vi "FTW-CodeGen-FindGObjectTaggedForScripting.vi"(0 "GObject to Traverse":refnum<vi>, 5 "Class Name":string="GObject", 7 "Label to uniquely identify node":string="#FTW-CodeGen", 11 "error in":errorcluster) -> (6 "GObject":refnum<vi>, 15 "error out":errorcluster)   [LabVIEW 2013, in "Featherweight.lvlib" / "FTW-CodeGen.lvlib"]
uses:
  FTW-CodeGen.lvlib
  Featherweight.lvlib
panel:
  # "Inputs"
  # "Outputs"
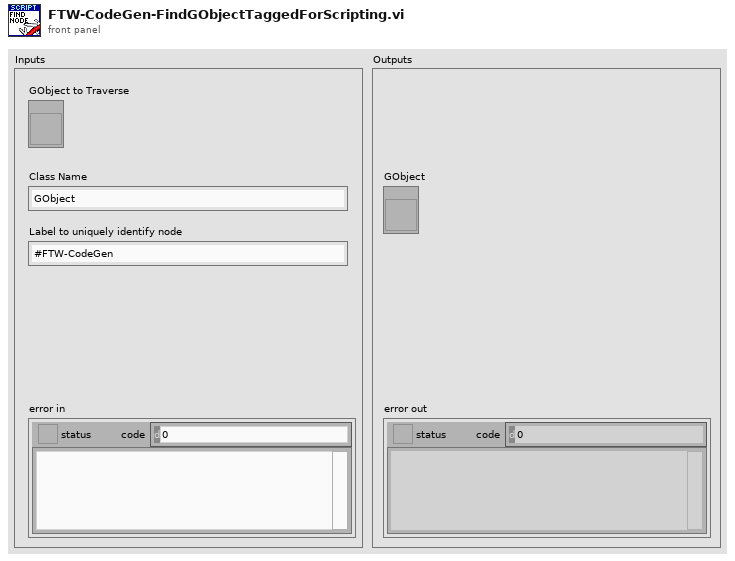
[diagram p1: front panel]
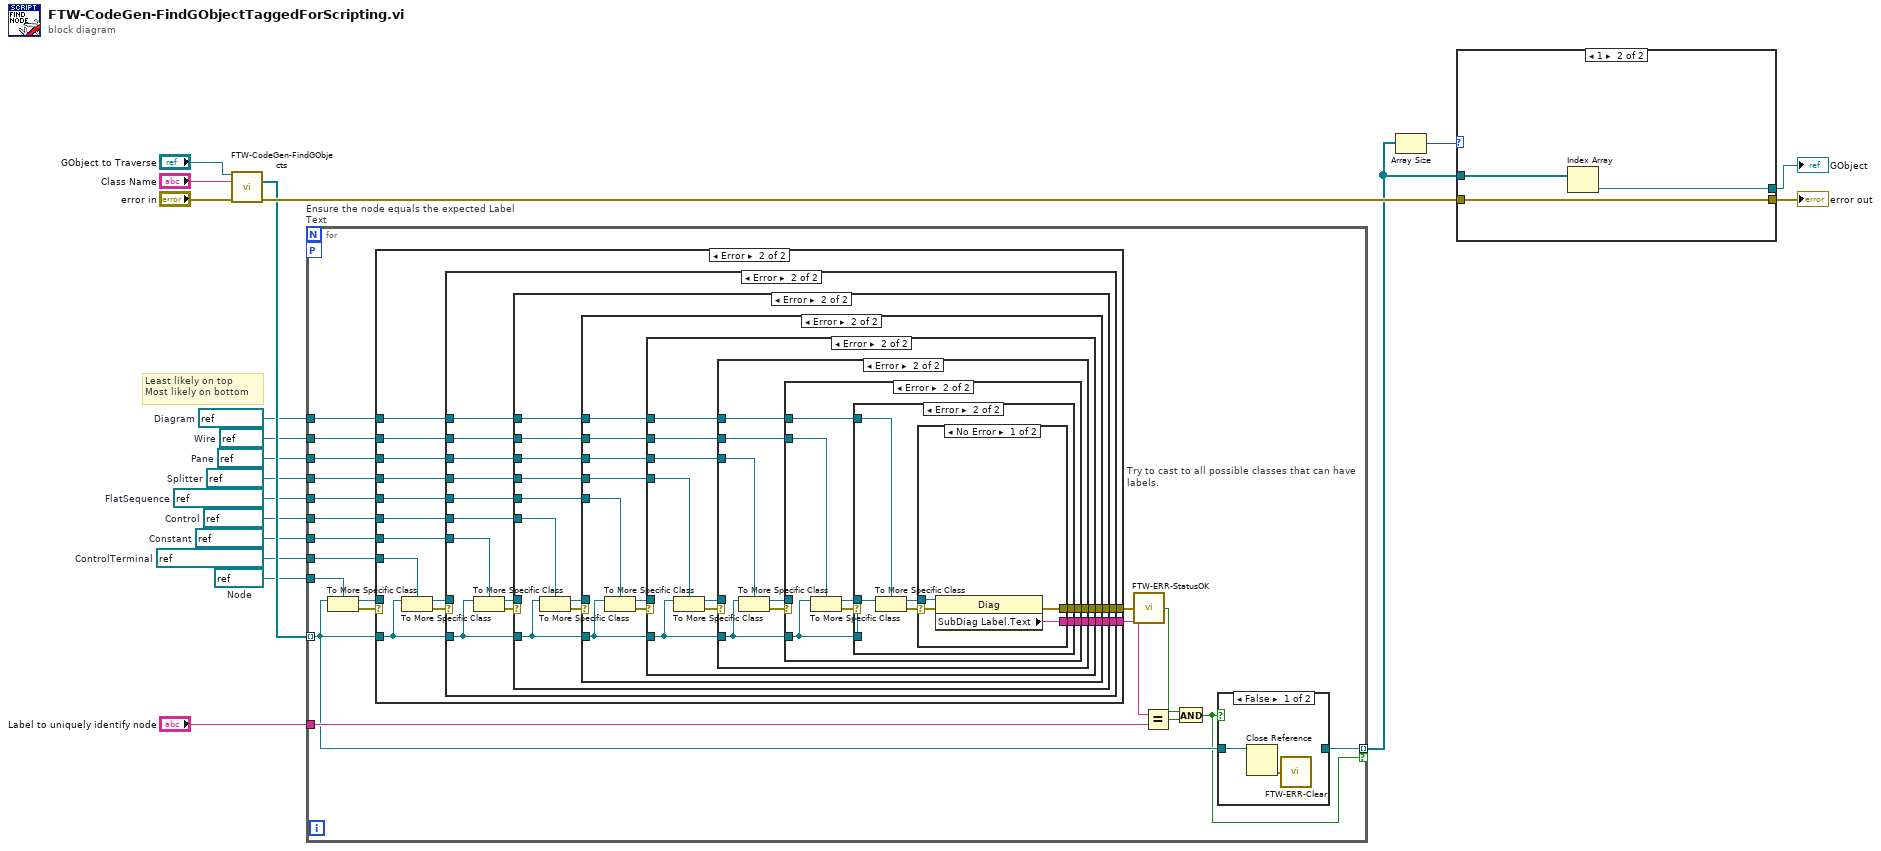
[diagram p0: block diagram]
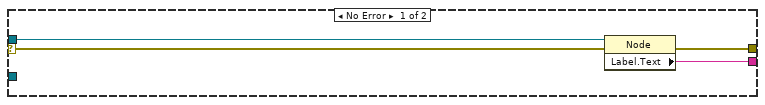
[diagram p3: hidden frame]
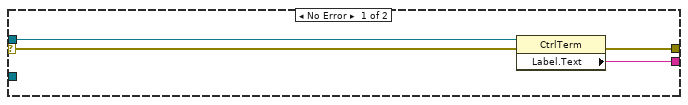
[diagram p4: hidden frame]
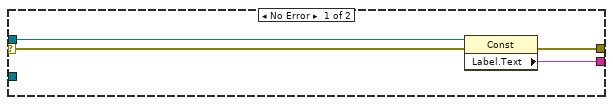
[diagram p5: hidden frame]
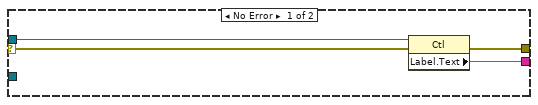
[diagram p6: hidden frame]
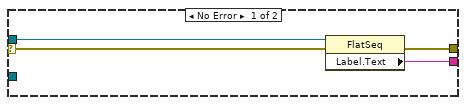
[diagram p7: hidden frame]
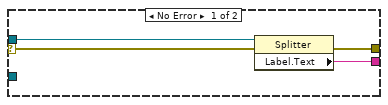
[diagram p8: hidden frame]
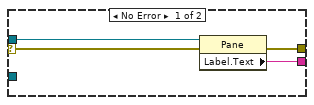
[diagram p9: hidden frame]
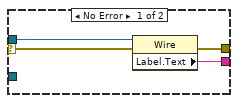
[diagram p10: hidden frame]
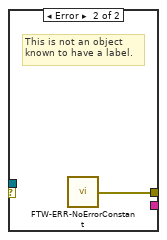
[diagram p11: hidden frame]
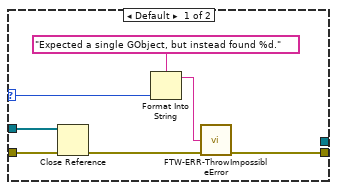
[diagram p12: hidden frame]
diagram:
  w3 = refnum<vi> refnum  # Constant
  w2 = refnum<vi> refnum  # ControlTerminal
  w4 = refnum<vi> refnum  # Control
  w5 = refnum<vi> refnum  # FlatSequence
  w6 = refnum<vi> refnum  # Splitter
  w7 = refnum<vi> refnum  # Pane
  w8 = refnum<vi> refnum  # Wire
  w9 = refnum<vi> refnum  # Diagram
  w1 = refnum<vi> refnum  # Node
  # "Least likely on top\nMost likely on bottom"
  n1 = call "FTW-CodeGen-FindGObjects.vi"("GObject to Traverse"="GObject to Traverse", "Class Name"="Class Name", "error in"="error in") -> ("GObject Instances"=w12:refnum<vi>[], "error out"=w14:errorcluster)  [unwired: 11 in]
  n2 = for "Ensure the node equals the expected Label Text" {
    tunnel: w12 -> [w22] mode=indexing
    tunnel: [w21] -> w11 mode=indexing if=w20
    workers-P: _ -> [_]
    tunnel: "Label to uniquely identify node" -> [w23]
    tunnel: w9 -> [w32]
    tunnel: w8 -> [w31]
    tunnel: w7 -> [w30]
    tunnel: w6 -> [w29]
    tunnel: w5 -> [w28]
    tunnel: w4 -> [w27]
    tunnel: w3 -> [w26]
    tunnel: w2 -> [w25]
    tunnel: w1 -> [w24]
    n3 = To More Specific Class(target class=w24, reference=w22) -> (specific class reference=w34:refnum<vi>, error out=w33:errorcluster)  [unwired: 1 in]
    n4 = case "Try to cast to all possible classes that can have labels." shown="Error" w33 {
      selector: w33 -> [w45 _]
      tunnel: w22 -> [_ w56]
      tunnel: w34 -> [w44 _]
      tunnel: [w43 w55] -> w35
      tunnel: [w42 w54] -> w37
      tunnel: w32 -> [_ w53]
      tunnel: w31 -> [_ w52]
      tunnel: w30 -> [_ w51]
      tunnel: w29 -> [_ w50]
      tunnel: w28 -> [_ w49]
      tunnel: w27 -> [_ w48]
      tunnel: w26 -> [_ w47]
      tunnel: w25 -> [_ w46]
      frame No Error {
        n5 = property class="Node"(reference=w44, error in=w45) -> (error out=w43:errorcluster, "Label.Text"=w42:string)  [unwired: 1 out]
      }
      frame Error {
        n6 = To More Specific Class(target class=w46, reference=w56) -> (specific class reference=w57:refnum<vi>, error out=w58:errorcluster)  [unwired: 1 in]
        n7 = case shown="Error" w58 {
          selector: w58 -> [w62 _]
          tunnel: w57 -> [w61 _]
          tunnel: w56 -> [_ w72]
          tunnel: [w60 w71] -> w55
          tunnel: [w59 w70] -> w54
          tunnel: w53 -> [_ w69]
          tunnel: w52 -> [_ w68]
          tunnel: w51 -> [_ w67]
          tunnel: w50 -> [_ w66]
          tunnel: w49 -> [_ w65]
          tunnel: w48 -> [_ w64]
          tunnel: w47 -> [_ w63]
          frame No Error {
            n8 = property class="CtrlTerm"(reference=w61, error in=w62) -> (error out=w60:errorcluster, "Label.Text"=w59:string)  [unwired: 1 out]
          }
          frame Error {
            n9 = To More Specific Class(target class=w63, reference=w72) -> (specific class reference=w73:refnum<vi>, error out=w74:errorcluster)  [unwired: 1 in]
            n10 = case shown="Error" w74 {
              selector: w74 -> [w78 _]
              tunnel: w73 -> [w77 _]
              tunnel: w72 -> [_ w87]
              tunnel: [w76 w86] -> w71
              tunnel: [w75 w85] -> w70
              tunnel: w69 -> [_ w84]
              tunnel: w68 -> [_ w83]
              tunnel: w67 -> [_ w82]
              tunnel: w66 -> [_ w81]
              tunnel: w65 -> [_ w80]
              tunnel: w64 -> [_ w79]
              frame No Error {
                n11 = property class="Const"(reference=w77, error in=w78) -> (error out=w76:errorcluster, "Label.Text"=w75:string)  [unwired: 1 out]
              }
              frame Error {
                n12 = To More Specific Class(target class=w79, reference=w87) -> (specific class reference=w88:refnum<vi>, error out=w89:errorcluster)  [unwired: 1 in]
                n13 = case shown="Error" w89 {
                  selector: w89 -> [w93 _]
                  tunnel: w88 -> [w92 _]
                  tunnel: w87 -> [_ w100]
                  tunnel: [w91 w101] -> w86
                  tunnel: [w90 w99] -> w85
                  tunnel: w84 -> [_ w98]
                  tunnel: w83 -> [_ w97]
                  tunnel: w82 -> [_ w96]
                  tunnel: w81 -> [_ w95]
                  tunnel: w80 -> [_ w94]
                  frame No Error {
                    n14 = property class="Ctl"(reference=w92, error in=w93) -> (error out=w91:errorcluster, "Label.Text"=w90:string)  [unwired: 1 out]
                  }
                  frame Error {
                    n15 = To More Specific Class(target class=w94, reference=w100) -> (specific class reference=w102:refnum<vi>, error out=w103:errorcluster)  [unwired: 1 in]
                    n16 = case shown="Error" w103 {
                      selector: w103 -> [w107 _]
                      tunnel: w102 -> [w106 _]
                      tunnel: [w105 w113] -> w101
                      tunnel: w100 -> [_ w115]
                      tunnel: [w104 w112] -> w99
                      tunnel: w98 -> [_ w111]
                      tunnel: w97 -> [_ w110]
                      tunnel: w96 -> [_ w109]
                      tunnel: w95 -> [_ w108]
                      frame No Error {
                        n17 = property class="FlatSeq"(reference=w106, error in=w107) -> (error out=w105:errorcluster, "Label.Text"=w104:string)  [unwired: 1 out]
                      }
                      frame Error {
                        n18 = To More Specific Class(target class=w108, reference=w115) -> (specific class reference=w114:refnum<vi>, error out=w116:errorcluster)  [unwired: 1 in]
                        n19 = case shown="Error" w116 {
                          selector: w116 -> [w118 _]
                          tunnel: w115 -> [_ w124]
                          tunnel: w114 -> [w120 _]
                          tunnel: [w119 w127] -> w113
                          tunnel: [w117 w125] -> w112
                          tunnel: w111 -> [_ w123]
                          tunnel: w110 -> [_ w122]
                          tunnel: w109 -> [_ w121]
                          frame No Error {
                            n20 = property class="Splitter"(reference=w120, error in=w118) -> (error out=w119:errorcluster, "Label.Text"=w117:string)  [unwired: 1 out]
                          }
                          frame Error {
                            n21 = To More Specific Class(target class=w121, reference=w124) -> (specific class reference=w126:refnum<vi>, error out=w128:errorcluster)  [unwired: 1 in]
                            n22 = case shown="Error" w128 {
                              selector: w128 -> [w132 _]
                              tunnel: [w130 w136] -> w127
                              tunnel: w126 -> [w131 _]
                              tunnel: [w129 w139] -> w125
                              tunnel: w124 -> [_ w135]
                              tunnel: w123 -> [_ w134]
                              tunnel: w122 -> [_ w133]
                              frame No Error {
                                n23 = property class="Pane"(reference=w131, error in=w132) -> (error out=w130:errorcluster, "Label.Text"=w129:string)  [unwired: 1 out]
                              }
                              frame Error {
                                n24 = To More Specific Class(target class=w133, reference=w135) -> (specific class reference=w137:refnum<vi>, error out=w138:errorcluster)  [unwired: 1 in]
                                n25 = case shown="Error" w138 {
                                selector: w138 -> [w142 _]
                                tunnel: [w140 w149] -> w139
                                tunnel: w137 -> [w143 _]
                                tunnel: [w141 w145] -> w136
                                tunnel: w135 -> [_ w148]
                                tunnel: w134 -> [_ w144]
                                frame No Error {
                                n26 = property class="Wire"(reference=w143, error in=w142) -> (error out=w141:errorcluster, "Label.Text"=w140:string)  [unwired: 1 out]
                                }
                                frame Error {
                                n27 = To More Specific Class(target class=w144, reference=w148) -> (specific class reference=w146:refnum<vi>, error out=w147:errorcluster)  [unwired: 1 in]
                                n28 = case shown="No Error" w147 {
                                selector: w147 -> [w150 _]
                                tunnel: [w151 _] -> w149
                                tunnel: w146 -> [w153 _]
                                tunnel: [w152 w154] -> w145
                                frame No Error {
                                n29 = property class="Diag"(reference=w153, error in=w150) -> (error out=w152:errorcluster, "SubDiag Label.Text"=w151:string)  [unwired: 1 out]
                                }
                                frame Error {
                                # "This is not an object\nknown to have a label."
                                n30 = call "FTW-ERR-NoErrorConstant.vi"() -> ("no error"=w154:errorcluster)
                                }
                                }
                                }
                                }
                              }
                            }
                          }
                        }
                      }
                    }
                  }
                }
              }
            }
          }
        }
      }
    }
    n31 = call "FTW-ERR-StatusOK.vi"("error to check"=w35) -> ("Status OK?"=w38:bool)
    n32 = Equal?(x=w37, y=w23) -> (x = y?=w36:bool)
    n33 = And(x=w38, y=w36) -> (x .and. y?=w20:bool)
    n34 = case shown="False" w20 {
      tunnel: [_ w41] -> w21
      tunnel: w22 -> [w40 w41]
      frame False {
        n35 = Close Reference(reference=w40) -> (error out=w39:errorcluster)  [unwired: 1 in]
        n36 = call "FTW-ERR-Clear.vi"("error to snuff"=w39) -> ()  [unwired: 1 out]
      }
      frame True {
      }
    }
  }
  n37 = Array Size(array=w11) -> (size(s)=w16:i32)
  n38 = case shown="1" w16 {
    selector: w16 -> [w159 _]
    tunnel: [w161 w164] -> w15
    tunnel: w14 -> [w156 w164]
    tunnel: w11 -> [w157 w163]
    tunnel: [_ w162] -> w13
    frame Default {
      n39 = Close Reference(reference=w157, error in (no error)=w156) -> (error out=w155:errorcluster)
      n40 = Format Into String(format string="Expected a single GObject, but instead found %d." ("Reason this error should never happen"), w159) -> (resulting string=w158:string)  [unwired: 2 in, 1 out]
      n41 = call "FTW-ERR-ThrowImpossibleError.vi"("Reason this error should never happen"=w158, "error in"=w155) -> ("error out"=w161:errorcluster)  [unwired: 13 in]
    }
    frame 1 {
      n42 = Index Array(array=w163) -> (element=w162:refnum<vi>)  [unwired: 1 in]
    }
  }
  "error out" <- w15
  "GObject" <- w13
